vi "StopMovement Core.vi"(8 "error in (no error)":errorcluster, 10 "AxisNumber":u8, 11 "CS++Nanotec in":refnum<class "CS++Nanotec.lvclass">) -> (0 "error out":errorcluster, 3 "CS++Nanotec out":refnum<class "CS++Nanotec.lvclass">)   [LabVIEW 2015, in "CS++Nanotec.lvlib" / "CS++Nanotec.lvclass"]
doc: "Stops the movement of an axis."
uses:
  CS++Nanotec.lvclass
  CS++Nanotec.lvclass/CS++Nanotec.ctl
  instr.lib/NanotecSMCPD/NanotecSMCPDDriver.lvlib
  CSPP_DeviceBase/CS++Motor/CS++Motor.lvclass
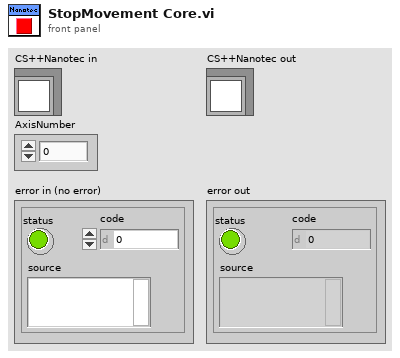
[diagram p1: front panel]
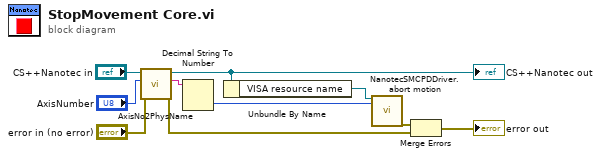
[diagram p0: block diagram]
diagram:
  n1 = call "AxisNo2PhysName.vi"("error in (no error)"="error in (no error)", "AxisNumber"="AxisNumber", "CS++Motor in"="CS++Nanotec in") -> ("error out"=w3:errorcluster, "PhysicalChannelName"=w2:string, "CS++Motor out"=w5:refnum<class "CS++Nanotec.lvclass">)  [unwired: 6 in]
  "CS++Nanotec out" <- w5
  n2 = Decimal String To Number(string=w2) -> (number=w1:i32)  [unwired: 2 in, 1 out]
  n3 = Unbundle By Name(w5) -> ("VISA resource name"=w8:refnum<visa-resource-name>)
  n4 = call "NanotecSMCPDDriver.abort motion.vi"("VISA resource name"=w8, "contollerID"=w1) -> ("error out"=w10:errorcluster)  [unwired: 15 in, 2 out]
  n5 = Merge Errors(w10, w3) -> (→"error out":errorcluster)
